vi "Create quad.vi"(0 "V0":sgl[](array[numeric]), 1 "V1":sgl[](array[numeric]), 2 "V2":sgl[](array[numeric]), 3 "V3":sgl[](array[numeric]), 4 "Plane":T1) -> (5 "Quad":T2)   [LabVIEW 2014]
uses:
  Typedefs/Quad.ctl
  Typedefs/Quadplane enum.ctl
  Dot product.vi
panel:
  # "PN 17/01/2015, 25/03/2015"
  # "Vertices"
  # "Edges"
  # "Unit normal"
  # "Plane ident."
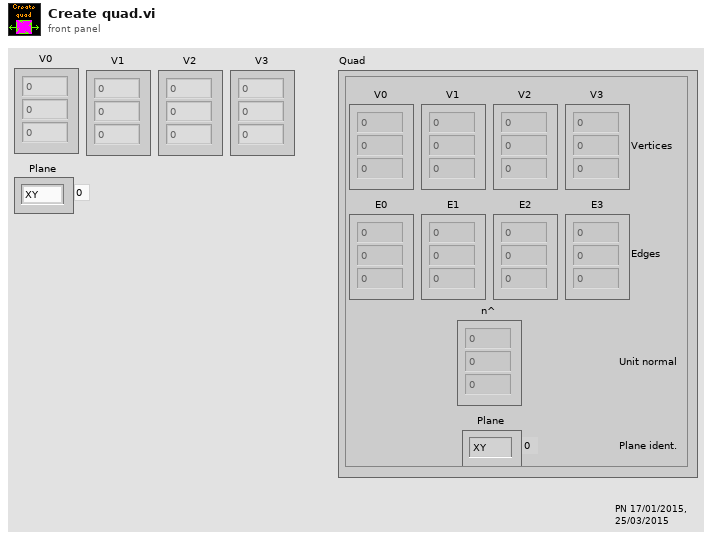
[diagram p1: front panel]
types:
  T1 = typedef "Quadplane enum.ctl" = enum8{"XY", "XZ", "YZ", "-XY", "-XZ", "-YZ"}
  T2 = typedef "Quad.ctl" = cluster{"V0":sgl[], "V1":sgl[], "V2":sgl[], "V3":sgl[], "E0":sgl[], "E1":sgl[], "E2":sgl[], "E3":sgl[], "n^":sgl[], "Plane":T1}
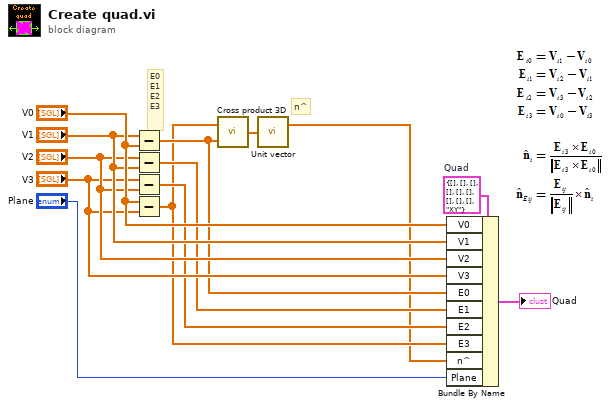
[diagram p0: block diagram]
diagram:
  w12 = T2 {"V0"=[], "V1"=[], "V2"=[], "V3"=[], "E0"=[], "E1"=[], "E2"=[], "E3"=[], "n^"=[], "Plane"=enum."XY"}  # Quad
  # "n^"
  # "E0\nE1\nE2\nE3"
  n1 = Subtract(x="V1", y="V0") -> (x-y=w7:sgl[])
  n2 = Subtract(x="V2", y="V1") -> (x-y=w6:sgl[])
  n3 = Subtract(x="V3", y="V2") -> (x-y=w5:sgl[])
  n4 = Subtract(x="V0", y="V3") -> (x-y=w4:sgl[])
  n5 = call "Cross product 3D.vi"("B"=w7, "A"=w4) -> ("A x B"=w13:sgl[])
  n6 = call "Unit vector.vi"("Vector"=w13) -> ("Unit vector"=w3:sgl[])  [unwired: 1 out]
  n7 = Bundle By Name(cluster=w12, "V0"="V0", "V1"="V1", "V2"="V2", "V3"="V3", "E0"=w7, "E1"=w6, "E2"=w5, "E3"=w4, "n^"=w3, "Plane"="Plane") -> (→"Quad":T2)
